vi "Auto_calibrate.vi"(3 "Mode":T4, 5 "Traverse line":T5 {"Row Duration (mins)" format="%#.1f"; "Row No" min=0; "Trace Gas Concentration (%)" min=0.0 format="%#.2f"; "Emission Rate (l/min)" format="%#.2f"; "Tunnel Speed" format="%#.2f"; "Start X" format="%#.2f"; "Start Y" format="%#.2f"; "Start Z" format="%#.2f"; "End X" format="%#.2f"; "End Y" format="%#.2f"; "End Z" format="%#.2f"; "Averaging time (min)" min=0.0 format="%#.2f"}) -> (0 "Error Messages":string, 1 "Status":T2, 2 "Traverse Out":T5 {"Row Duration (mins)" format="%#.1f"; "Row No" min=0; "Trace Gas Concentration (%)" min=0.0 format="%#.2f"; "Emission Rate (l/min)" format="%#.2f"; "Tunnel Speed" format="%#.2f"; "Start X" format="%#.2f"; "Start Y" format="%#.2f"; "Start Z" format="%#.2f"; "End X" format="%#.2f"; "End Y" format="%#.2f"; "End Z" format="%#.2f"; "Averaging time (min)" min=0.0 format="%#.2f"})   [LabVIEW 2012]
uses:
  Gen Trav/Traverse_cluster.ctl
  Gen Trav/Spacing.ctl
  Controls/Multi_run_mode.ctl
  Controls/User_Specific_mode.ctl
  Controls/Auto_Calib_Type.ctl
  Gen Trav/Multi_Run_Status.ctl
  Controls/Auto_Calib_Case.ctl
  File/Setup_Filetype.ctl
  Calibration/Calib_mode.ctl
  Controls/Setup.ctl
  Controls/Post_Process.ctl
  Controls/Save_Data.ctl
  Controls/App_Global.ctl
  Globals/Meas_global.vi
  Globals/Calib_global.vi
  Globals/Trav_pos_global.vi
  <vilib>/Analysis/baseanly.llb/Mean (DBL).vi
  Globals/Extra_Commands_Global.vi
  <vilib>/Analysis/NI_AALBase.lvlib
panel:
  out "Minimum St Dev":dbl[](array[numeric])
  out "Time FFID valve moved":dbl
  out "Wait factor":dbl
  out "Establishment time":string
  out "Orig Calib file string":string
  out "Concentrations":dbl[](array[numeric])
  out "FFID St Dev":dbl[][](array[numeric]) format="%.2f"
  in  "Clear Calib History":bool
  out "Coefficients":dbl[][](array[numeric]) format="%.2f"
  out "Currently in Case":T1
  out "Valve position":dbl format="%.2f"
  out "Currently On":i32
  out "Values":dbl[][](array[numeric]) format="%.2f"
  out "FF Indexes":i16[](array[numeric])
  out "Ch No's":i16[](array[numeric])
  out "No of Calib Points":i32
  out "Root Name":string[](array[string])
  out "Original Calib File":path
  out "Calibration varying":T3
  in  "stop":bool
  out "New Calib Filenames":path[](array[path])
  # "Specific Argument Options\n      Tunnel Speed;1;2;3;4\nOR  Traverse Position\nOR   Concentration"
  # "X           Y            Z"
  # "Start"
  # "End"
  # "X           Y            Z"
  # "Start"
  # "End"
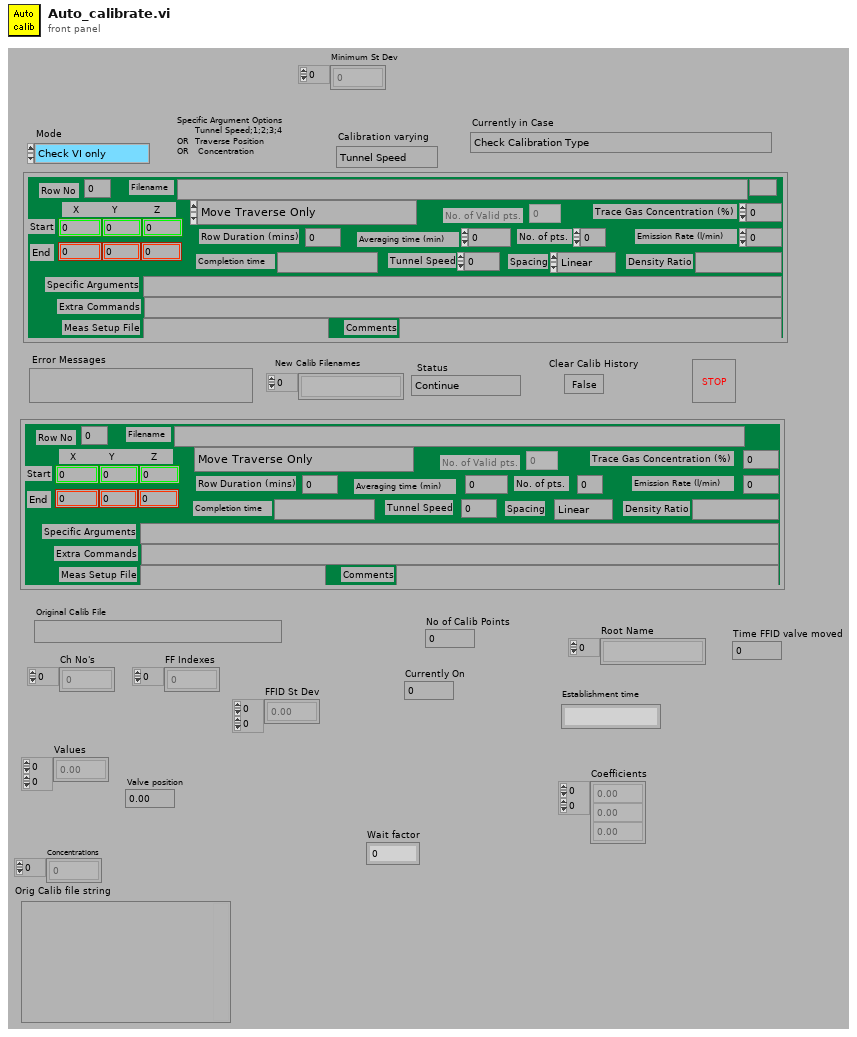
[diagram p1: front panel]
types:
  T1 = typedef "Auto_Calib_Case.ctl" = enum16{"Check Calibration Type", "Check if Original Calib file is Valid", "Get sampling rate etc. from meas setup file", "Setup Calibration Program", "Get Channel Numbers", "Check use latest selected on Mesurement setup files", "Create New Calib Filenames", "Setup Calibration Values in 2D array", "Create Measurement Setup File (Concentration Only)", "Are There Enough Calibration Points", "Set Measurement Conditions", "Measure Calibration Point", "Do Another Calibration Point?", "Skip Next Frame?", "Insert New calibration Filenames into Measurement Setup file", "Warn if FFID calibration is very non linear", "Warn if FFID variance is high", "Insert Bkgnd Variance into calib file", "Warn if FFID voltages are too low", "Warn if Current Calibration fit is poor", "Warn if Calibration Coefficients have significantly altered", "End"}
  T2 = typedef "Multi_Run_Status.ctl" = enum16{"Continue", "Jump to Next Point", "Jump to Next Row", "Jump To Fall Back", "Terminate Run"}
  T3 = typedef "Auto_Calib_Type.ctl" = enum16{"Tunnel Speed", "Traverse Position", "Concentration"}
  T4 = typedef "User_Specific_mode.ctl" = enum16{"Check VI only", "Run VI"}
  T5 = typedef "Traverse_cluster.ctl" = cluster{"Start X":dbl, "Start Y":dbl, "Start Z":dbl, "End X":dbl, "End Y":dbl, "End Z":dbl, "No. of pts.":i32, "Spacing":T6, "Filename":path, "Tunnel Speed":dbl, "Averaging time (min)":dbl, "Extra Commands":string, "Specific Arguments":string, "Emission Rate (l/min)":dbl, "Trace Gas Concentration (%)":dbl, "Density Ratio":string, "Comments":string, "Row No":i32, "Row Type Selector":T7, "Completion time":string, "Row Duration (mins)":dbl, "No. of Valid pts.":i32, "Meas Setup File":string}
  T6 = typedef "Spacing.ctl" = enum16{"Linear", "Log", "Gauss", "Specified", "N/A"}
  T7 = typedef "Multi_run_mode.ctl" = enum16{"Move Traverse Only", "Set Tunnel Speed Only", "Set Source Only", "Set Measurement Conditions", "Single Measurement", "Vertical Profile", "Lateral Profile", "Longitudinal Profile", "Explore Volume", "Multi-Axis Profile", "Auto Calibrate", "Meas Fast FID Bkgnd", "Check Beam Power", "Scanning Valve Measurement", "Run VI Named:", "Set ADAM Ch", "Wait (minutes)", "Send Message", "Synchronize With:", "Fall Back to this Row", "Turn Off Row Repeating", "Blank Row", "Traverse 3D Volume"}
  T8 = typedef "Setup_Filetype.ctl" = enum16{"Measurement Setups", "Calibration Setups", "General", "Results File Plotter Setups", "Speed Calib Tweaks"}
  T9 = typedef "Calib_mode.ctl" = enum16{"Show Setup", "Take a New Calibration Point", "Refit Curve", "Setup Front Panel"}
  T10 = typedef "Save_Data.ctl" = enum16{"Save No Data", "Save Data"}
  T11 = typedef "Post_Process.ctl" = enum16{"Take New Data", "Post Process Raw Data File"}
  T12 = typedef "Setup.ctl" = enum16{"Run Program", "Show Setup", "Save Current Setup", "Setup Front Panel"}
  T13 = typedef "App_Global.ctl" = enum16{"Read Global", "Write to Global", "Initialise Array"}
  T14 = typedef "Cal_Inst_type.ctl" = enum16{"Propeller anemometer", "Pressure Transducer", "Hot wire", "Cross wire velocity", "Cross wire angle", "Generic Linear", "Generic Polynomial", "Generic BackPoly", "Fast FID", "Thermocouple", "Cold wire", "Pulsed Wire"}
  T15 = typedef "Ref_Inst_type.ctl" = enum16{"Propellor anemometer", "Pressure Transducer", "Raw voltage", "Pitot-static tube", "Preston tube", "Generic Linear", "Generic Polynomial", "Thermocouple", "LDA", "Enter Value", "ADAM Channel"}
  T16 = cluster{"2nd Ref type":T15, "2nd inst present":bool}
  T17 = cluster{"high limit (10V)":sgl, "low limit (-10V)":sgl, "Ch No":i16, "Var name":string}[]
  T18 = cluster{"high limit (10V)":sgl, "low limit (-10V)":sgl, "Ch No":i16, "Var name":string}
  T19 = typedef "Inst_type.ctl" = enum16{"Propeller anemometer", "Raw voltage", "Pressure Transducer", "Pitot-static tube", "Preston tube", "Hot wire", "Cross wire 1", "Cross wire 2", "Generic Linear", "Generic Polynomial", "Generic BackPoly", "Fast FID", "Thermocouple", "Cold wire", "Pulsed Wire", "LDA Vel", "LDA Tran time", "LDA Arr time"}
  T20 = cluster{"high limit (10V)":sgl, "low limit (-10V)":sgl, "Ch No":i16, "Calib filename":path, "Inst type":T19, "Symbol":string, "Move channel":bool, "Use Latest":bool, "D":dbl, "Ch Name":string}[]
  T21 = typedef "Status_Cluster.ctl" = cluster{"Status":T2, "Error Type":string, "Error Description":string}
  T22 = typedef "Valco_valve_ph.ctl" = u16
  T23 = typedef "Time_Trace_Cluster.ctl" = cluster{"Weighting":dbl[], "Time (s)":dbl[], "Voltage":dbl[], "Eng Values":dbl[]}
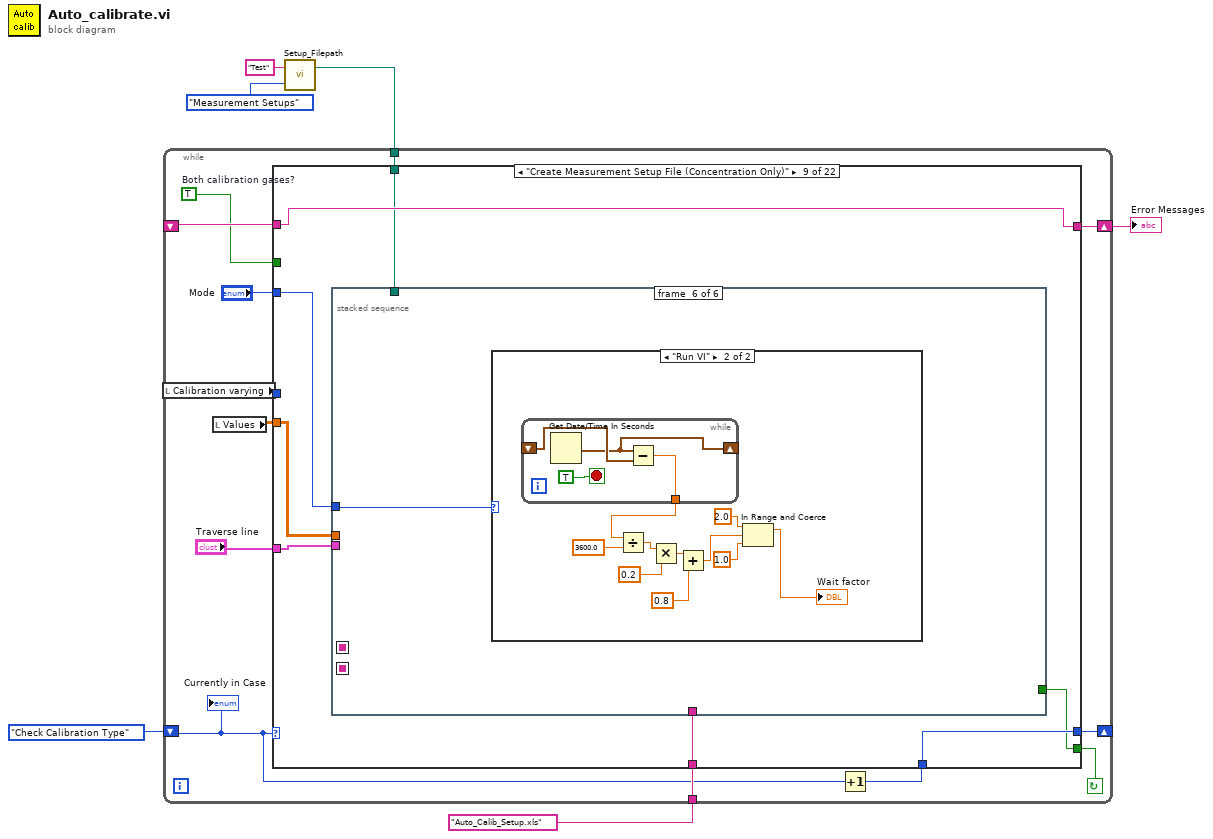
[diagram p0: block diagram]
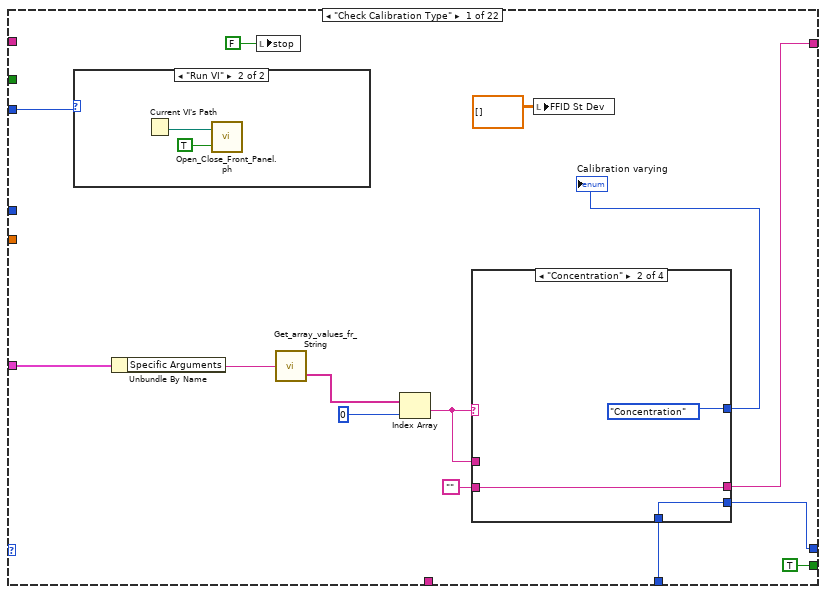
[diagram p2: hidden frame]
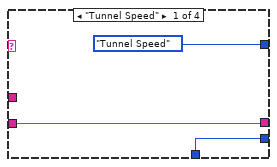
[diagram p4: hidden frame]
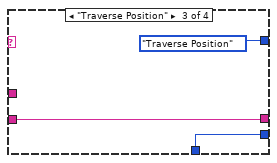
[diagram p5: hidden frame]
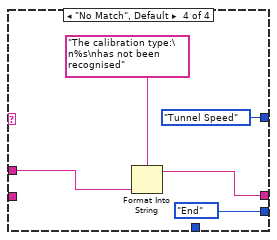
[diagram p6: hidden frame]
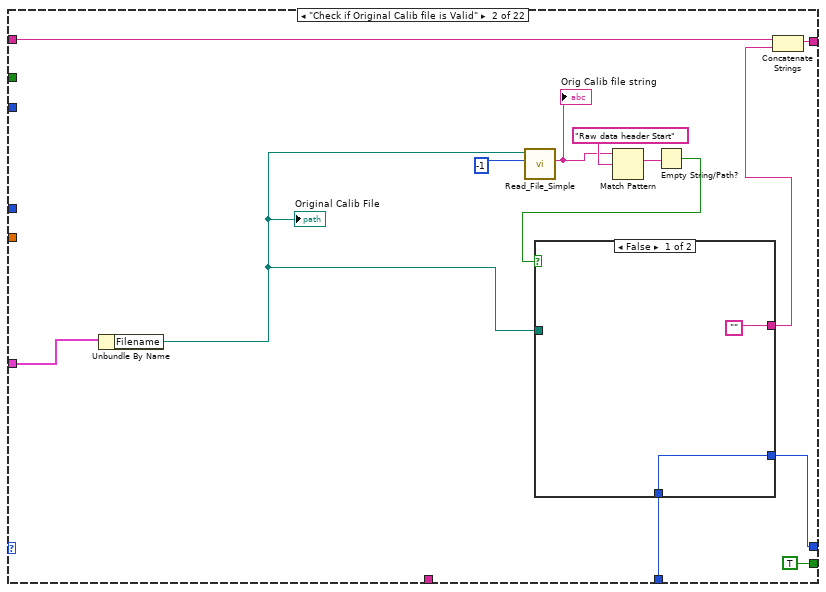
[diagram p7: hidden frame]
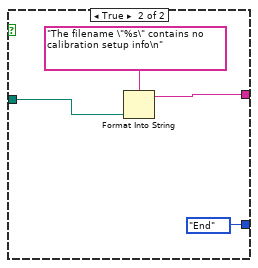
[diagram p8: hidden frame]
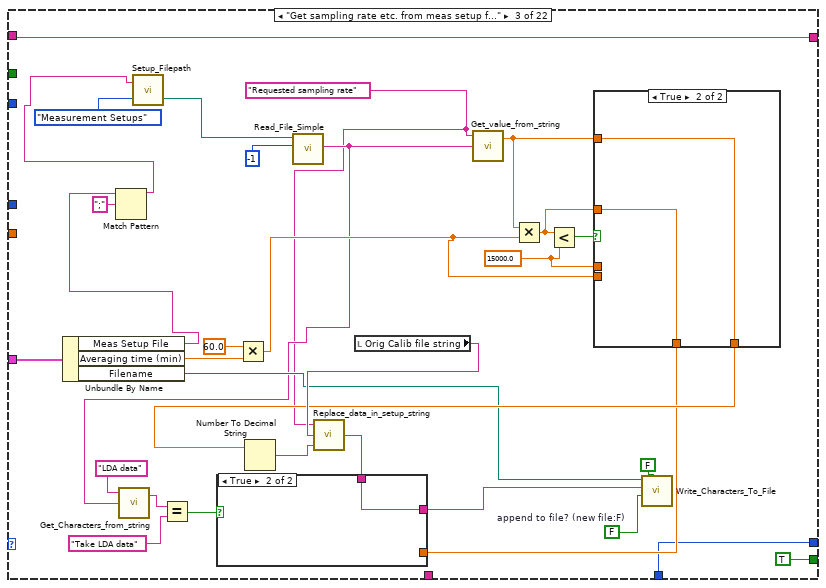
[diagram p9: hidden frame]
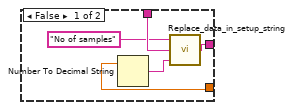
[diagram p10: hidden frame]
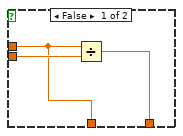
[diagram p11: hidden frame]
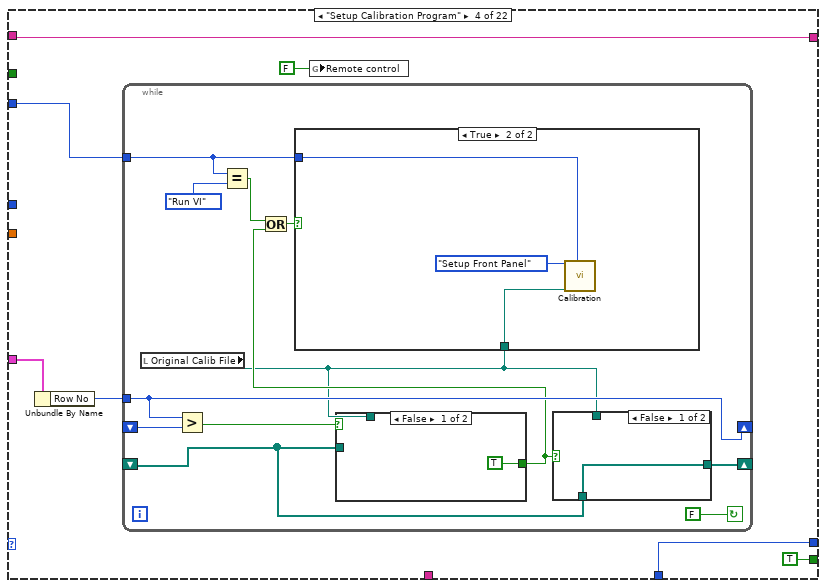
[diagram p12: hidden frame]
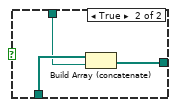
[diagram p13: hidden frame]
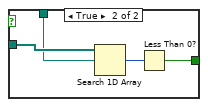
[diagram p15: hidden frame]
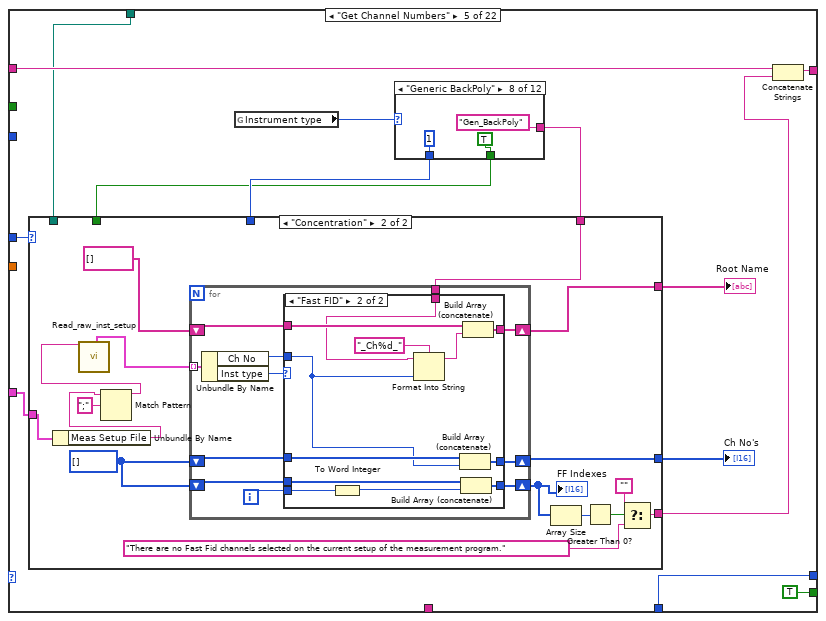
[diagram p16: hidden frame]
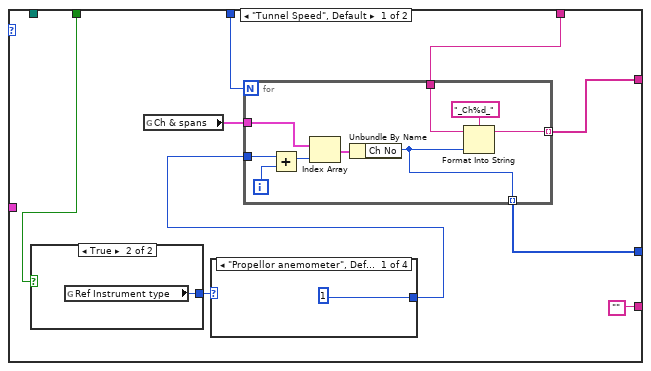
[diagram p17: hidden frame]
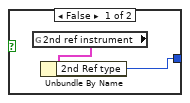
[diagram p18: hidden frame]
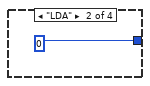
[diagram p19: hidden frame]
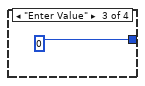
[diagram p20: hidden frame]
diagram:
  n1 = call "Setup_Filepath.vi"("Setup File Type"=Setup_Filetype."Measurement Setups", "Filename in"="Test") -> ("Directory"=w1:path)  [unwired: 1 out]
  n2 = while {
    shift-left: _ -> [w11]
    shift-right: [w12] -> w5
    shift-left: Auto_Calib_Case."Check Calibration Type" ("Currently in Case") -> [w10]
    shift-right: [w9] -> _
    tunnel: "Auto_Calib_Setup.xls" -> [w19]
    tunnel: w1 -> [w7]
    stop <- w15 continue-if-true
    w8 = TRUE  # Both calibration gases?
    n3 = local read "Calibration varying"() -> (w14:T3)
    n4 = local read "Values"() -> (w13:dbl[][])
    n5 = Increment(x=w10) -> (x+1=w16:T1)
    n6 = case shown="\"Create Measurement Setup File (Concentration Only)\"" w10 {
      tunnel: "Traverse line" -> [w33 w62 w100 w114 w145 _ _ w367 w400 _ w553 _ _ _ _ _ _ _ _ _ w970 w1001]
      tunnel: "Mode" -> [w24 _ _ w115 _ _ w318 _ w401 _ w548 _ w714 _ _ _ _ _ _ _ _ w1002]
      tunnel: w19 -> [_ _ _ _ _ _ _ _ w405 _ _ w625 _ _ _ _ _ _ _ _ _ _]
      tunnel: [w22 w52 w82 w117 w148 w264 w315 w358 w403 w516 w541 w624 w715 w741 w753 w772 w810 w875 w893 w949 w993 w1007] -> w9
      tunnel: w16 -> [w23 w51 w82 w117 w148 w264 w315 w359 w403 w515 w535 w624 _ w740 w752 w772 w810 w875 w893 w949 w993 w1007]
      tunnel: [TRUE TRUE TRUE TRUE TRUE TRUE TRUE TRUE w399 TRUE TRUE TRUE TRUE TRUE TRUE TRUE TRUE TRUE TRUE TRUE TRUE FALSE] -> w15
      tunnel: w14 -> [_ _ _ _ w152 _ w314 w365 _ _ w539 w626 w713 w739 w755 _ _ _ _ _ _ w1003]
      tunnel: w13 -> [_ _ _ _ _ _ _ _ w398 w525 w552 _ _ _ _ _ w817 _ w899 _ _ _]
      tunnel: [w26 w54 w80 w118 w149 w265 w329 w362 w404 w519 w536 w622 w712 w744 w759 w781 w824 w871 w900 w938 w986 w1006] -> w12
      tunnel: w11 -> [_ w56 w80 w118 w151 w265 w329 w361 w404 w520 w536 w622 w712 w744 w759 w781 w824 w871 w900 w938 w986 w1006]
      tunnel: w8 -> [_ _ _ _ _ _ _ w360 _ _ _ _ _ _ _ _ _ _ _ _ _ w1000]
      tunnel: w7 -> [_ _ _ _ w144 w267 _ _ w402 _ _ _ _ _ _ _ _ _ _ _ _ _]
      frame "Check Calibration Type" {
        n7 = case shown="\"Run VI\"" w24 {
          frame "Check VI only" {
          }
          frame "Run VI" {
            n8 = Current VI's Path() -> (path=w34:path)
            n9 = call "Open_Close_Front_Panel.ph.vi"("Front Panel Window:Open"=TRUE, "VI path"=w34) -> ()  [unwired: 2 out]
          }
        }
        n10 = Unbundle By Name(w33) -> ("Specific Arguments"=w32:string)
        n11 = local write "stop"(FALSE) -> ()
        n12 = call "Get_array_values_fr_String.vi"("String Value"=w32) -> ("String array"=w31:string[])  [unwired: 1 out]
        n13 = Index Array(array=w31, index=0 ("Index")) -> (element=w29:string)
        n14 = case shown="\"Concentration\"" w29 {
          tunnel: [Auto_Calib_Type."Tunnel Speed" ("Calibration varying") Auto_Calib_Type."Concentration" ("Calibration varying") Auto_Calib_Type."Traverse Position" ("Calibration varying") Auto_Calib_Type."Tunnel Speed" ("Calibration varying")] -> w27
          tunnel: w29 -> [_ _ _ w48]
          tunnel: [w37 w40 w43 w46] -> w26
          tunnel: "" -> [w37 w40 w43 _]
          tunnel: w23 -> [w36 w39 w42 _]
          tunnel: [w36 w39 w42 Auto_Calib_Case."End" ("Currently in Case")] -> w22
          frame "Tunnel Speed" {
          }
          frame "Concentration" {
            (unwired) ""
          }
          frame "Traverse Position" {
          }
          frame "No Match", Default {
            n15 = Format Into String(format string="The calibration type:\n%s\nhas not been recognised" ("Format String"), w48) -> (resulting string=w46:string)  [unwired: 2 in, 1 out]
          }
        }
        "Calibration varying" <- w27
        n16 = local write "FFID St Dev"(dbl[][] [] ("FFID Variance")) -> ()
      }
      frame "Check if Original Calib file is Valid" {
        n17 = Unbundle By Name(w62) -> ("Filename"=w50:path)
        "Original Calib File" <- w50
        n18 = call "Read_File_Simple.vi"("Filename"=w50, "number of characters (all:-1)"=-1) -> ("string"=w59:string)  [unwired: 1 in, 7 out]
        "Orig Calib file string" <- w59
        n19 = Match Pattern(string=w59, regular expression="Raw data header Start") -> (match substring=w58:string)  [unwired: 4 out]
        n20 = Empty String/Path?(string/path=w58) -> (empty?=w57:bool)
        n21 = case shown="False" w57 {
          tunnel: w50 -> [_ w68]
          tunnel: ["" w66] -> w55
          tunnel: [w63 Auto_Calib_Case."End" ("Currently in Case")] -> w52
          tunnel: w51 -> [w63 _]
          frame False {
          }
          frame True {
            n22 = Format Into String(format string="The filename \"%s\" contains no calibration setup info\n" ("Format String"), w68) -> (resulting string=w66:string)  [unwired: 2 in, 1 out]
          }
        }
        n23 = Concatenate Strings(w56, w55) -> (w54:string)
      }
      frame "Get sampling rate etc. from meas setup file" {
        w83 = FALSE  # append to file? (new file:F)
        w72 = "Requested sampling rate"
        w90 = 15000.0 ("y")
        n24 = Unbundle By Name(w100) -> ("Meas Setup File"=w78:string, "Averaging time (min)"=w98:dbl, "Filename"=w85:path)
        n25 = Match Pattern(string=w78, regular expression=";") -> (before substring=w70:string)  [unwired: 4 out]
        n26 = call "Setup_Filepath.vi"("Setup File Type"=Setup_Filetype."Measurement Setups", "Filename in"=w70) -> ("Filename Out"=w69:path)  [unwired: 1 out]
        n27 = Multiply(x=60.0, y=w98) -> (x*y=w89:dbl)
        n28 = call "Read_File_Simple.vi"("Filename"=w69, "number of characters (all:-1)"=-1) -> ("string"=w77:string)  [unwired: 1 in, 7 out]
        n29 = call "Get_Characters_from_string.vi"("Input string"=w77, "Variable name"="LDA data") -> ("Value"=w75:string)  [unwired: 1 in, 1 out]
        n30 = Equal?(x=w75, y="Take LDA data") -> (x = y?=w73:bool)
        n31 = local read "Orig Calib file string"() -> (w94:string)
        n32 = call "Get_value_from_string.vi"("Input string"=w77, "Variable name"=w72) -> ("Value"=w93:dbl)  [unwired: 1 in, 1 out]
        n33 = Multiply(x=w93, y=w89) -> (x*y=w88:dbl)
        n34 = Less?(x=w88, y=w90) -> (x < y?=w96:bool)
        n35 = case shown="True" w96 {
          tunnel: w93 -> [_ w111]
          tunnel: [w108 w111] -> w92
          tunnel: w90 -> [w107 _]
          tunnel: w89 -> [w109 _]
          tunnel: [w107 w110] -> w86
          tunnel: w88 -> [_ w110]
          frame False {
            n36 = Divide(x=w107, y=w109) -> (x/y=w108:dbl)
          }
          frame True {
          }
        }
        n37 = Number To Decimal String(number=w92) -> (decimal integer string=w91:string)  [unwired: 1 out]
        n38 = call "Replace_data_in_setup_string.vi"("New data string"=w91, "Input string"=w94, "Variable name"=w72) -> ("Appended string"=w87:string)
        n39 = case shown="True" w73 {
          tunnel: w87 -> [w105 w106]
          tunnel: w86 -> [w102 _]
          tunnel: [w101 w106] -> w84
          frame False {
            n40 = Number To Decimal String(number=w102) -> (decimal integer string=w103:string)  [unwired: 1 out]
            n41 = call "Replace_data_in_setup_string.vi"("New data string"=w103, "Input string"=w105, "Variable name"="No of samples") -> ("Appended string"=w101:string)
          }
          frame True {
          }
        }
        n42 = call "Write_Characters_To_File.vi"("file path (dialog if empty)"=w85, "advisory dialog? (display:T)"=FALSE, "character string"=w84, "append to file? (new file:F)"=w83) -> ()  [unwired: 1 in, 4 out]
      }
      frame "Setup Calibration Program" {
        n43 = Unbundle By Name(w114) -> ("Row No"=w113:i32)
        n44 = while {
          shift-left: _ -> [w122]
          shift-right: [w120] -> _
          tunnel: w113 -> [w129]
          shift-left: _ -> [w130]
          shift-right: [w129] -> _
          tunnel: w115 -> [w127]
          stop <- FALSE continue-if-true
          n45 = local read "Original Calib File"() -> (w121:path)
          n46 = Greater?(x=w129, y=w130) -> (0:w128:bool)
          n47 = Equal?(x=w127, y=User_Specific_mode."Run VI" ("Mode")) -> (x = y?=w125:bool)
          n48 = case shown="False" w128 {
            tunnel: w122 -> [_ w142]
            tunnel: w121 -> [_ w141]
            tunnel: [TRUE w139] -> w123
            frame False {
            }
            frame True {
              n49 = Search 1D Array(1D array=w142, element=w141) -> (index of element=w140:i32)  [unwired: 1 out]
              n50 = Less Than 0?(x=w140) -> (x < 0?=w139:bool)
            }
          }
          n51 = Or(x=w125, y=w123) -> (x .or. y?=w124:bool)
          n52 = case shown="True" w124 {
            tunnel: w127 -> [_ w137]
            tunnel: w121 -> [_ w136]
            frame False {
            }
            frame True {
              n53 = call "Calibration.vi"("Mode"=Calib_mode."Setup Front Panel", "Calib file"=w136, "Simulate/Run"=w137) -> ()  [unwired: 17 out]
            }
          }
          n54 = case shown="False" w123 {
            tunnel: w122 -> [w131 w134]
            tunnel: w121 -> [_ w133]
            tunnel: [w131 w132] -> w120
            frame False {
            }
            frame True {
              n55 = Build Array (concatenate)(w134, w133) -> (w132:path[])
            }
          }
        }
        n56 = global write "Meas_global.vi" "Remote control"(FALSE ("Remote control")) -> ()
      }
      frame "Get Channel Numbers" {
        n57 = global read "Calib_global.vi" "Instrument type"() -> (w156:T14)
        n58 = case shown="\"Generic BackPoly\"" w156 {
          tunnel: ["Prop" "Mano" "HW" "XW" "XW" "Gen_Lin" "Gen_Poly" "Gen_BackPoly" "FF" "Therm" "CW" "PWA"] -> w155
          tunnel: [1 1 1 2 2 1 1 1 1 1 1 1] -> w146
          tunnel: [TRUE TRUE TRUE TRUE FALSE TRUE TRUE TRUE TRUE TRUE TRUE TRUE] -> w143
          frame "Propeller anemometer" {
          }
          frame "Pressure Transducer" {
          }
          frame "Hot wire" {
          }
          frame "Cross wire velocity" {
          }
          frame "Cross wire angle" {
          }
          frame "Generic Linear" {
          }
          frame "Generic Polynomial" {
          }
          frame "Generic BackPoly" {
          }
          frame "Fast FID" {
          }
          frame "Thermocouple" {
          }
          frame "Cold wire" {
          }
          frame "Pulsed Wire" {
          }
        }
        n59 = case shown="\"Concentration\"" w152 {
          tunnel: w155 -> [w163 w197]
          tunnel: [w159 w196] -> w154
          tunnel: [w160 w194] -> w153
          tunnel: ["" w187] -> w150
          tunnel: w146 -> [w161 _]
          tunnel: w145 -> [_ w186]
          tunnel: w144 -> [_ _]
          tunnel: w143 -> [w157 _]
          frame "Tunnel Speed", Default {
            n60 = case shown="True" w157 {
              tunnel: [w166 w168] -> w165
              frame False {
                n61 = global read "Calib_global.vi" "2nd ref instrument"() -> (w167:T16)
                n62 = Unbundle By Name(w167) -> ("2nd Ref type"=w166:T15)
              }
              frame True {
                n63 = global read "Calib_global.vi" "Ref Instrument type"() -> (w168:T15)
              }
            }
            n64 = global read "Calib_global.vi" "Ch & spans"() -> (w162:T17)
            n65 = case shown="\"Propellor anemometer\", Default" w165 {
              tunnel: [1 i16 0 0 0] -> w158
              frame "Propellor anemometer", Default {
              }
              frame "LDA" {
              }
              frame "Enter Value" {
              }
              frame "ADAM Channel" {
              }
            }
            n66 = for {
              N: w161 -> [_]
              tunnel: [w175] -> w160 mode=indexing
              tunnel: w163 -> [w174]
              tunnel: w162 -> [w173]
              tunnel: [w172] -> w159 mode=indexing
              tunnel: w158 -> [w170]
              i -> [w171]
              n67 = Add(x=w170, y=w171) -> (x+y=w169:i32)
              n68 = Index Array(array=w173, index=w169) -> (element=w177:T18)
              n69 = Unbundle By Name(w177) -> ("Ch No"=w175:i16)
              n70 = Format Into String(format string="_Ch%d_" ("Format String"), initial string=w174, w175) -> (resulting string=w172:string)  [unwired: 1 in, 1 out]
            }
          }
          frame "Concentration" {
            w193 = i16[] []
            n71 = Unbundle By Name(w186) -> ("Meas Setup File"=w183:string)
            n72 = Match Pattern(string=w183, regular expression=";") -> (before substring=w182:string)  [unwired: 4 out]
            n73 = call "Read_raw_inst_setup.vi"("Setup file"=w182) -> ("Ch & spans choices"=w185:T20)  [unwired: 18 out]
            n74 = for {
              tunnel: w185 -> [w208] mode=indexing
              tunnel: w197 -> [w207]
              shift-right: [w203] -> w196
              shift-left: string[] [] -> [w204]
              shift-right: [w201] -> w194
              shift-left: w193 -> [w202]
              shift-right: [w200] -> w192
              shift-left: w193 -> [w199]
              i -> [w198]
              n75 = Unbundle By Name(w208) -> ("Ch No"=w206:i16, "Inst type"=w205:T19)
              n76 = case shown="\"Fast FID\"" w205 {
                tunnel: w207 -> [_ w213]
                tunnel: w206 -> [_ w215]
                tunnel: w204 -> [w211 w223]
                tunnel: [w211 w222] -> w203
                tunnel: w202 -> [w210 w221]
                tunnel: [w210 w220] -> w201
                tunnel: w199 -> [w209 w218]
                tunnel: [w209 w219] -> w200
                tunnel: w198 -> [_ w217]
                frame "Generic Linear", Default {
                }
                frame "Fast FID" {
                  n77 = To Word Integer(number=w217) -> (16bit integer=w216:i16)
                  n78 = Format Into String(format string="_Ch%d_", initial string=w213, w215) -> (resulting string=w212:string)  [unwired: 1 in, 1 out]
                  n79 = Build Array (concatenate)(w221, w215) -> (w220:i16[])
                  n80 = Build Array (concatenate)(w218, w216) -> (w219:i16[])
                  n81 = Build Array (concatenate)(w223, w212) -> (w222:string[])
                }
              }
            }
            "FF Indexes" <- w192
            n82 = Array Size(array=w192) -> (size(s)=w191:i32)
            n83 = Greater Than 0?(x=w191) -> (x > 0?=w190:bool)
            n84 = Select(t="", s=w190, f="There are no Fast Fid channels selected on the current setup of the measurement program.") -> (s? t:f=w187:string)
          }
        }
        "Root Name" <- w154
        "Ch No's" <- w153
        n85 = Concatenate Strings(w151, w150) -> (w149:string)
      }
      frame "Check use latest selected on Mesurement setup files" {
        n86 = global read "Trav_pos_global.vi" "Measurement setup files"() -> (w260:string[])
        n87 = local read "Ch No's"() -> (w266:i16[])
        n88 = Build Array (concatenate)(w260, "Current_Setup.xls") -> (w261:string[])
        n89 = for {
          tunnel: w267 -> [w270]
          tunnel: w261 -> [w269] mode=indexing
          tunnel: w266 -> [w268]
          n90 = stacked-sequence {
            seq-local: [w271 _ _] -> [_ w277 w305]
            seq-local: [_ w275 _] -> [_ _ w303]
            tunnel: w270 -> [w274 _ w302]
            tunnel: w269 -> [w273 _ w301]
            tunnel: w268 -> [_ w276 _]
            frame #0 {
              n91 = Build Path(base path=w274, name or relative path=w273) -> (appended path=w272:path)
              n92 = call "Read_File_Simple.vi"("Filename"=w272) -> ("string"=w271:string)  [unwired: 2 in, 7 out]
            }
            frame #1 {
              n93 = while {
                shift-right: [w282] -> w275
                shift-left: w277 -> [w283]
                tunnel: w276 -> [w286]
                i -> [w290]
                stop <- w279 continue-if-true
                n94 = Increment(x=w290) -> (x+1=w284:i32)
                n95 = Format Into String(format string="An ch %d Ch No", w284) -> (resulting string=w289:string)  [unwired: 2 in, 1 out]
                n96 = call "Get_value_from_string.vi"("Input string"=w283, "Variable name"=w289) -> ("Status"=w288:enum16{"Char in string", "Char not in string"}, "Value"=w287:dbl)  [unwired: 1 in]
                n97 = To Long Integer(number=w287) -> (32bit integer=w285:i32)
                n98 = Search 1D Array(1D array=w286, element=w285) -> (index of element=w281:i32)  [unwired: 1 in]
                n99 = Greater Or Equal To 0?(x=w281) -> (x >= 0?=w280:bool)
                n100 = case shown="\"Char in string\"" w288 {
                  tunnel: [TRUE FALSE] -> w279
                  frame "Char in string" {
                  }
                  frame "Char not in string" {
                  }
                }
                n101 = And(x=w280, y=w279) -> (x .and. y?=w278:bool)
                n102 = case shown="True" w278 {
                  tunnel: w284 -> [w294 _]
                  tunnel: w283 -> [w293 w298]
                  tunnel: [w292 w298] -> w282
                  frame True {
                    n103 = Format Into String(format string="An ch %d Use latest Calib", w294) -> (resulting string=w296:string)  [unwired: 2 in, 1 out]
                    n104 = call "Replace_data_in_setup_string.vi"("New data string"="TRUE" ("Replace with"), "Input string"=w293, "Variable name"=w296) -> ("Appended string"=w292:string)
                  }
                  frame False {
                  }
                }
              }
            }
            frame #2 {
              n105 = Equal?(x=w305, y=w303) -> (x = y?=w304:bool)
              n106 = case shown="True" w304 {
                tunnel: w302 -> [w308 _]
                tunnel: w303 -> [w311 _]
                tunnel: w301 -> [w307 _]
                frame False {
                  w310 = FALSE  # append to file? (new file:F)
                  n107 = Build Path(base path=w308, name or relative path=w307) -> (appended path=w306:path)
                  n108 = call "Write_Characters_To_File.vi"("file path (dialog if empty)"=w306, "advisory dialog? (display:T)"=FALSE, "character string"=w311, "append to file? (new file:F)"=w310) -> ()  [unwired: 1 in, 4 out]
                }
                frame True {
                }
              }
            }
          }
        }
      }
      frame "Create New Calib Filenames" {
        n109 = local read "Original Calib File"() -> (w327:path)
        n110 = Get Date/Time String(date format (0)=enum16{"short", "long", "abbreviated"}."short") -> (date string=w322:string)  [unwired: 3 out]
        n111 = Strip Path(path=w327) -> (stripped path=w317:path)  [unwired: 1 out]
        n112 = local read "Root Name"() -> (w313:string[])
        n113 = case shown="\"Tunnel Speed\", Default" w314 {
          tunnel: w313 -> [_ w334]
          tunnel: [1 w333] -> w312
          frame "Tunnel Speed", Default {
          }
          frame "Concentration" {
            n114 = Array Size(array=w334) -> (size(s)=w333:i32)
          }
        }
        n115 = call "Replace_Character.vi"("Replace with"="-", "Input String"=w322, "Search For"="/") -> ("Output string"=w319:string)  [unwired: 1 out]
        n116 = List Folder(path=w317) -> (filenames=w331:string[])  [unwired: 1 in, 5 out]
        n117 = To Upper Case(1:w331) -> (0:w330:string[])
        n118 = for {
          N: w312 -> [_]
          tunnel: w313 -> [w337] mode=indexing
          tunnel: w330 -> [w341]
          tunnel: w317 -> [w340]
          tunnel: [w336] -> w326 mode=indexing
          tunnel: w319 -> [w338]
          tunnel: w318 -> [w335]
          n119 = while {
            tunnel: w337 -> [w348]
            tunnel: w338 -> [w349]
            tunnel: [w344] -> w339
            tunnel: w341 -> [w351]
            i -> [w353]
            stop <- w355 continue-if-true
            n120 = Increment(x=w353) -> (x+1=w350:i32)
            n121 = Format Into String(format string="%s_%d.xls" ("Format String"), initial string=w348, w349, w350) -> (resulting string=w345:string)  [unwired: 1 in, 1 out]
            n122 = call "Replace_Character.vi"("Replace with"="_", "Input String"=w345, "Search For"=" ") -> ("Output string"=w344:string)  [unwired: 1 out]
            n123 = To Upper Case(1:w344) -> (0:w354:string)
            n124 = Search 1D Array(1D array=w351, element=w354) -> (index of element=w356:i32)  [unwired: 1 out]
            n125 = Not Equal?(x=w356, y=-1) -> (x != y?=w355:bool)
          }
          n126 = Build Path(base path=w340, name or relative path=w339) -> (appended path=w336:path)
          n127 = case shown="\"Run VI\"" w335 {
            tunnel: w336 -> [_ w342]
            frame "Check VI only" {
            }
            frame "Run VI" {
              n128 = call "Calibration.vi"("Mode"=Calib_mode."Setup Front Panel", "Calib file"=w342) -> ()  [unwired: 1 in, 17 out]
            }
          }
        }
        "New Calib Filenames" <- w326
        n129 = Index Array(array=w326, index=0 ("Index")) -> (element=w324:path)
        n130 = global write "Meas_global.vi" "Results file"(w324) -> ()
        "Establishment time" <- "!Establish Exp Conditions (s) = 15" ("Message")
      }
      frame "Setup Calibration Values in 2D array" {
        n131 = case shown="\"Concentration\"" w365 {
          tunnel: [w376 w382 w397] -> w364
          tunnel: w367 -> [w371 _ w396]
          tunnel: ["" "" w395] -> w363
          tunnel: w360 -> [_ w380 _]
          tunnel: w359 -> [w370 w379 w394]
          tunnel: [w369 w379 w393] -> w358
          frame "Tunnel Speed" {
            n132 = Unbundle By Name(w371) -> ("Specific Arguments"=w374:string)
            n133 = call "Get_array_values_fr_String.vi"("String Value"=w374) -> ("Numeric Array"=w372:dbl[])  [unwired: 1 out]
            n134 = Array Subset(array=w372, index=1 ("Array Index")) -> (w368:dbl[])  [unwired: 1 in]
            n135 = for {
              tunnel: w368 -> [w378] mode=indexing
              tunnel: [w377] -> w376 mode=indexing
              n136 = Build Array(w378) -> (w377:dbl[])
            }
            n137 = Increment(x=w370) -> (x+1=w369:T1)
          }
          frame "Concentration" {
            n138 = case shown="True" w380 {
              tunnel: [w384 w388] -> w383
              frame True {
                n139 = Build Array(3.0, 2.0, 1.0) -> (w384:dbl[])
              }
              frame False {
                n140 = Build Array(1.0, 3.0) -> (w388:dbl[])
              }
            }
            n141 = for {
              tunnel: w383 -> [w392] mode=indexing
              tunnel: [w391] -> w382 mode=indexing
              n142 = Build Array(w392) -> (w391:dbl[])
            }
          }
          frame "Traverse Position" {
            n143 = call "Create_Pos_array.vi"("Traverse line"=w396) -> ("Error Messages"=w395:string, "Array of Positions"=w397:dbl[][])  [unwired: 5 in, 2 out]
            n144 = Increment(x=w394) -> (x+1=w393:T1)
          }
        }
        "Values" <- w364
        n145 = Concatenate Strings(w361, w363) -> (w362:string)
      }
      frame "Create Measurement Setup File (Concentration Only)" {
        n146 = stacked-sequence {
          seq-local: [w416 _ _ _ _ _] -> [_ w435 _ _ _ _]
          seq-local: [_ w433 _ _ _ _] -> [_ _ w456 _ _ _]
          tunnel: w402 -> [w407 _ w457 _ _ _]
          tunnel: w405 -> [_ _ w458 _ _ _]
          tunnel: w401 -> [_ _ _ w464 w483 w500]
          tunnel: w400 -> [w413 _ _ _ w484 _]
          tunnel: [_ _ _ _ w482 _] -> w399
          tunnel: w398 -> [_ _ _ w467 _ _]
          frame #0 {
            w420 = TRUE  # Show Dialog?
            n147 = Unbundle By Name(w413) -> ("Meas Setup File"=w414:string)
            n148 = Match Pattern(string=w414, regular expression=";") -> (before substring=w412:string)  [unwired: 4 out]
            n149 = Build Path(base path=w407, name or relative path=w412) -> (appended path=w421:path)
            n150 = Format Into String(format string="Meas Setup File   %s", w407) -> (resulting string=w406:string)  [unwired: 2 in, 1 out]
            n151 = call "Read_spec_No_of_Characters.vi"("Filename"=w421) -> ("character string"=w422:string)  [unwired: 1 out]
            n152 = call "Get_string_subset.vi"("String Name"=w406, "Show Dialog?"=w420, "String to split"=w422, "File Label"="Raw data header") -> ("Output string"=w409:string)  [unwired: 1 out]
            n153 = call "Get_value_from_string.vi"("Input string"=w409, "Variable name"="No of analogue inst") -> ("Value"=w410:dbl)  [unwired: 1 in, 1 out]
            n154 = for {
              N: w410 -> [_]
              shift-right: [w424] -> w419
              shift-left: w409 -> [w426]
              i -> [w430]
              n155 = Increment(x=w430) -> (x+1=w429:i32)
              n156 = Number To Decimal String(number=w429) -> (decimal integer string=w432:string)  [unwired: 1 out]
              n157 = Concatenate Strings("An ch ", w432, " Inst type") -> (w427:string)
              n158 = call "Replace_data_in_setup_string.vi"("New data string"="Raw voltage", "Input string"=w426, "Variable name"=w427) -> ("Appended string"=w424:string)
            }
            n159 = call "Replace_data_in_setup_string.vi"("New data string"="No LDA data", "Input string"=w419, "Variable name"="LDA data" ("Label for characters")) -> ("Appended string"=w416:string)
          }
          frame #1 {
            n160 = global read "Calib_global.vi" "New Setup String"() -> (w436:string)
            n161 = for {
              N: 4 -> [_]
              shift-right: [w441] -> w433
              shift-left: w435 -> [w442]
              tunnel: w436 -> [w438]
              i -> [w440]
              n162 = case shown="3" w440 {
                tunnel: [w445 w448 w451 "No of blocks"] -> w439
                tunnel: w438 -> [w444 w447 w450 _]
                tunnel: [w443 w446 w449 "1" ("Value")] -> w437
                frame 0, Default {
                  w445 = "No of samples"
                  n163 = call "Get_Characters_from_string.vi"("Input string"=w444, "Variable name"=w445) -> ("Value"=w443:string)  [unwired: 1 in, 1 out]
                }
                frame 2 {
                  w448 = "Actual sampling rate"
                  n164 = call "Get_Characters_from_string.vi"("Input string"=w447, "Variable name"=w448) -> ("Value"=w446:string)  [unwired: 1 in, 1 out]
                }
                frame 3 {
                  w451 = "Board type"
                  n165 = call "Get_Characters_from_string.vi"("Input string"=w450, "Variable name"=w451) -> ("Value"=w449:string)  [unwired: 1 in, 1 out]
                }
                frame 1 {
                }
              }
              n166 = call "Replace_data_in_setup_string.vi"("New data string"=w437, "Input string"=w442, "Variable name"=w439) -> ("Appended string"=w441:string)
            }
          }
          frame #2 {
            w462 = FALSE  # advisory dialog? (display:T)
            w463 = FALSE  # append to file? (new file:F)
            n167 = call "Remove_Plug_Ins_etc.vi"("Input String"=w456) -> ("Output string"=w455:string)
            n168 = call "Add_label_to_string.vi"("String to write"=w455, "File Label"="Raw data header") -> ("Output string"=w459:string)
            n169 = Build Path(base path=w457, name or relative path=w458) -> (appended path=w454:path)
            n170 = call "Add_length_to_string.vi"("String in"=w459) -> ("String out"=w461:string)
            n171 = call "Write_Characters_To_File.vi"("file path (dialog if empty)"=w454, "advisory dialog? (display:T)"=w462, "character string"=w461, "append to file? (new file:F)"=w463) -> ()  [unwired: 1 in, 4 out]
          }
          frame #3 {
            w466 = 0 ("Index")
            w471 = 0.0 ("Input Element")
            n172 = Index Array(array=w467, index (row)=w466, index (col)=w466) -> (element=w465:dbl)
            n173 = case shown="\"Run VI\"" w464 {
              tunnel: w465 -> [_ w474]
              frame "Check VI only" {
              }
              frame "Run VI" {
                n174 = flat-sequence {
                  tunnel: w474 -> [w475]
                  frame #0 {
                    n175 = call "Fast_FID_Valve_Control.vi"("Requested Position"=w475) -> ()  [unwired: 7 out]
                  }
                  frame #1 {
                    n176 = Get Date/Time In Seconds() -> (seconds since 1Jan1904=w477:timestamp)
                    n177 = To Double Precision Float(number=w477) -> (double precision float=→"Time FFID valve moved":dbl)
                  }
                }
              }
            }
            n178 = Build Array("GMU:Calibration:Gas 1", "GMU:Calibration:Gas 2") -> (w473:string[])
            n179 = call "Get_Current_Scan_client.vi"("ADAM Ch Names"=w473) -> ("Numerical Values"=w472:dbl[])  [unwired: 3 out]
            n180 = Build Array (concatenate)(w471, w471, w472, w471) -> (→"Concentrations":dbl[])
          }
          frame #4 {
            w481 = dbl[] [30.0, 15.0, 0.0] ("appended array")
            n181 = Unbundle By Name(w484) -> ("Start Z"=w478:dbl)
            n182 = Array Size(array=w481) -> (size(s)=w480:i32)
            n183 = Decrement(x=w480) -> (x-1=w479:i32)
            n184 = while {
              tunnel: w483 -> [w493]
              tunnel: w484 -> [w497]
              tunnel: w481 -> [w496] mode=indexing
              tunnel: w478 -> [w494]
              tunnel: w479 -> [w489]
              tunnel: [w485] -> w482
              i -> [w490]
              stop <- w486 continue-if-true
              n185 = Add(x=w494, y=w496) -> (x+y=w495:dbl)
              n186 = Less?(x=w490, y=w489) -> (x < y?=w487:bool)
              n187 = Bundle By Name(cluster=w497, "Start Z"=w495) -> (w498:T5)
              n188 = call "Set_Traverse_Position.vi"("Simulate/Run"=w493, "Currently on Point"=1, "Traverse line"=w498) -> ("Status Cluster"=w488:T21)  [unwired: 2 out]
              n189 = Unbundle By Name(w488) -> ("Status"=w491:T2)
              n190 = call "Prog_Status_Handler.vi"("Status Cluster"=w488, "Simulate/Run"=w493) -> ()  [unwired: 2 out]
              n191 = local write "Status"(w491) -> ()
              n192 = Equal?(x=w491, y=Multi_Run_Status."Continue" ("Status")) -> (x = y?=w485:bool)
              n193 = And(x=w485, y=w487) -> (x .and. y?=w486:bool)
            }
          }
          frame #5 {
            n194 = case shown="\"Run VI\"" w500 {
              frame "Check VI only", Default {
              }
              frame "Run VI" {
                n195 = while {
                  shift-right: [w512] -> _
                  shift-left: _ -> [w513]
                  tunnel: [w511] -> w506
                  stop <- TRUE stop-if-true
                  n196 = Get Date/Time In Seconds() -> (seconds since 1Jan1904=w512:timestamp)
                  n197 = Subtract(x=w512, y=w513) -> (x-y=w511:dbl)
                }
                n198 = Divide(x=w506, y=3600.0) -> (x/y=w505:dbl)
                n199 = Multiply(x=w505, y=0.2) -> (x*y=w503:dbl)
                n200 = Add(x=w503, y=0.8) -> (x+y=w501:dbl)
                n201 = In Range and Coerce(upper limit=2.0, x=w501, lower limit=1.0) -> (coerced(x)=→"Wait factor":dbl)  [unwired: 1 out]
              }
            }
          }
        }
      }
      frame "Are There Enough Calibration Points" {
        n202 = Array Size(array=w525) -> (size(s)=w526:i32[])
        n203 = Index Array(array=w526, index=0 ("Index")) -> (element=w521:i32)
        "No of Calib Points" <- w521
        n204 = Greater?(x=w521, y=1) -> (0:w522:bool)
        n205 = case shown="False" w522 {
          tunnel: ["Less than two calibration points have been specified\n" ""] -> w518
          tunnel: [Auto_Calib_Case."End" ("Currently in Case") w530] -> w516
          tunnel: w515 -> [_ w530]
          frame False {
          }
          frame True {
          }
        }
        n206 = Concatenate Strings(w520, w518) -> (w519:string)
        "Currently On" <- 1 ("Currently On")
      }
      frame "Set Measurement Conditions" {
        n207 = local read "Currently On"() -> (w540:i32)
        n208 = Decrement(x=w540) -> (x-1=w551:i32)
        n209 = Index Array(array=w552, index (row)=w551) -> (element=w550:dbl[])  [unwired: 1 in]
        n210 = case shown="\"Concentration\"" w539 {
          tunnel: w550 -> [w568 w585 w602]
          tunnel: w548 -> [_ _ w600]
          tunnel: w553 -> [w566 w581 w591]
          tunnel: [w567 w580 w589] -> w534
          tunnel: w540 -> [w562 _ w592]
          tunnel: [w565 w579 w596] -> w532
          frame "Tunnel Speed" {
            n211 = Index Array(array=w568, index=0 ("Index")) -> (element=w555:dbl)
            n212 = while {
              shift-right: [w576] -> w557
              shift-left: _ -> [w575]
              tunnel: w555 -> [w578]
              tunnel: [w576] -> w564
              tunnel: [w575] -> w563
              stop <- FALSE continue-if-true
              n213 = Greater Than 0?(x=w578) -> (x > 0?=w576:bool)
            }
            n214 = Exclusive Or(1:w563, 2:w564) -> (0:w560:bool)
            n215 = Greater?(x=w562, y=1) -> (0:w559:bool)
            n216 = And(x=w560, y=w559) -> (x .and. y?=w558:bool)
            n217 = case shown="False" w557 {
              tunnel: [w570 w572] -> w556
              tunnel: w555 -> [w571 w572]
              frame False {
                n218 = Negate(x=w571) -> (-x=w570:dbl)
              }
              frame True {
              }
            }
            n219 = case shown="True" w558 {
              frame False {
              }
              frame True {
                n220 = call "Wait_Seconds_with_display.vi"("Message"="Please rotate the probe you are calibrating", "Seconds to wait"=10000.0) -> ()  [unwired: 2 out]
              }
            }
            n221 = local read "Establishment time"() -> (w565:string)
            n222 = Bundle By Name(cluster=w566, "Tunnel Speed"=w556) -> (w567:T5)
          }
          frame "Traverse Position" {
            n223 = Index Array(array=w585, index=0 ("Index")) -> (element=w584:dbl)
            n224 = Index Array(array=w585, index=1 ("Index")) -> (element=w583:dbl)
            n225 = Index Array(array=w585, index=2 ("Index")) -> (element=w582:dbl)
            n226 = local read "Establishment time"() -> (w579:string)
            n227 = Bundle By Name(cluster=w581, "Start X"=w584, "Start Y"=w583, "Start Z"=w582) -> (w580:T5)
          }
          frame "Concentration" {
            w590 = nan ("Start X")
            n228 = local read "Wait factor"() -> (w595:dbl)
            n229 = Index Array(array=w602, index=0 ("Index")) -> (element=w593:dbl)
            n230 = case shown="1, Default" w592 {
              tunnel: [w604 w612 100.0] -> w594
              tunnel: w595 -> [w610 w613 _]
              frame 1, Default {
                n231 = local read "Time FFID valve moved"() -> (w607:dbl)
                n232 = Get Date/Time In Seconds() -> (seconds since 1Jan1904=w609:timestamp)
                n233 = Multiply(x=w610, y=35.0) -> (x*y=w606:dbl)
                n234 = To Double Precision Float(number=w609) -> (double precision float=w608:dbl)
                n235 = Subtract(x=w608, y=w607) -> (x-y=w605:dbl)
                n236 = Subtract(x=w606, y=w605) -> (x-y=w604:dbl)
              }
              frame 2 {
                n237 = Multiply(x=w613, y=25.0) -> (x*y=w612:dbl)
              }
              frame 3 {
              }
            }
            n238 = case shown="\"Check VI only\"" w600 {
              tunnel: w593 -> [w617 w618]
              tunnel: [w616 w619] -> w601
              frame "Check VI only" {
                n239 = To Long Integer(number=w617) -> (32bit integer=w616:i32)
              }
              frame "Run VI" {
                n240 = call "Fast_FID_Valve_Control.vi"("Requested Position"=w618) -> ("Achieved Posn."=w619:T22)  [unwired: 6 out]
              }
            }
            n241 = Number To Decimal String(number=w594) -> (decimal integer string=w597:string)  [unwired: 1 out]
            n242 = Concatenate Strings("!Establish Exp Conditions (s) = " ("Message"), w597) -> (w596:string)
            n243 = To Double Precision Float(number=w601) -> (double precision float=→"Valve position":dbl)
            n244 = Bundle By Name(cluster=w591, "Start X"=w590, "Start Y"=w590, "Start Z"=w590) -> (w589:T5)
          }
        }
        n245 = call "Add_Extra_Command.vi"("Traverse line"=w534, "Extra Command"=w532) -> ("Traverse line Out"=w533:T5)
        n246 = call "Set_Measurement_Conditions.vi"("Simulate/Run"=w548, "Currently on Point"=1, "Traverse line"=w533) -> ("Status Cluster"=w538:T21)  [unwired: 2 out]
        n247 = Unbundle By Name(w538) -> ("Status"=w537:T2)
        "Status" <- w537
        n248 = Equal?(x=w537, y=Multi_Run_Status."Continue" ("Status")) -> (x = y?=w544:bool)
        n249 = Equal?(x=User_Specific_mode."Run VI" ("Mode"), y=w548) -> (x = y?=w545:bool)
        n250 = Increment(x=w535) -> (x+1=w542:T1)
        n251 = And(x=w544, y=w545) -> (x .and. y?=w543:bool)
        n252 = Select(t=w535, s=w543, f=w542) -> (s? t:f=w541:T1)
      }
      frame "Measure Calibration Point" {
        n253 = case shown="\"Concentration\"" w626 {
          tunnel: w625 -> [_ w635]
          tunnel: [w629 w634] -> w621
          tunnel: [w627 w633] -> w620
          frame "Tunnel Speed", Default {
            n254 = local read "New Calib Filenames"() -> (w630:path[])
            n255 = Index Array(array=w630, index=0 ("Index")) -> (element=w631:path)
            n256 = call "Calibration.vi"("Mode"=Calib_mode."Take a New Calibration Point", "Calib file"=w631) -> ("Coefficients"=w627:dbl[][], "Status Out"=w629:T2)  [unwired: 1 in, 15 out]
          }
          frame "Concentration" {
            # "St Dev"
            # "Mean"
            n257 = stacked-sequence {
              seq-local: [_ w639 _] -> [_ _ w684]
              seq-local: [_ w638 _] -> [_ _ w683]
              tunnel: w635 -> [_ w642 _]
              tunnel: [_ w640 _] -> w634
              tunnel: [_ _ w685] -> w633
              frame #0 {
                n258 = global write "Meas_global.vi" "Remote control"(TRUE ("Remote control")) -> ()
                n259 = global write "Meas_global.vi" "Raw data option"(enum16{"Save raw data", "Raw data not saved"}."Save raw data" ("Raw data option")) -> ()
              }
              frame #1 {
                n260 = local read "New Calib Filenames"() -> (w643:path[])
                n261 = Index Array(array=w643, index=0 ("Index")) -> (element=w641:path)
                n262 = while {
                  tunnel: [w651] -> w640
                  tunnel: w641 -> [w650]
                  tunnel: w642 -> [w648]
                  tunnel: [w647] -> w639
                  tunnel: [w646] -> w638
                  i -> [w645]
                  stop <- w649 continue-if-true
                  n263 = stacked-sequence {
                    seq-local: [_ w653 _ _] -> [_ _ _ w677]
                    seq-local: [_ _ w662 _] -> [_ _ _ w681]
                    tunnel: [_ w653 _ _] -> w651
                    tunnel: w650 -> [_ w658 _ _]
                    tunnel: [_ _ _ w672] -> w649
                    tunnel: w648 -> [_ w654 _ _]
                    tunnel: [_ _ w663 _] -> w647
                    tunnel: [_ _ w662 _] -> w646
                    tunnel: w645 -> [_ _ _ w679]
                    frame #0 {
                      n264 = global write "Meas_global.vi" "Remote control"(TRUE ("Remote control")) -> ()
                    }
                    frame #1 {
                      n265 = call "Get_Data_Base_file_code.vi"("Results Filename"=w658, "Data Type"="Raw_Calibrations") -> ("Raw Data File Name"=w655:path)  [unwired: 3 out]
                      n266 = call "Measurement.vi"("setup"=Setup."Run Program", "Post Process"=Post_Process."Take New Data", "File"=Save_Data."Save No Data", "Raw data file"=w655, "Setup filename"=w654) -> ("Status Out"=w653:T2)  [unwired: 2 in, 12 out]
                    }
                    frame #2 {
                      n267 = local read "FF Indexes"() -> (w664:i16[])
                      n268 = global read "Meas_global.vi" "Time Trace"() -> (w661:T23[])
                      n269 = for {
                        tunnel: w664 -> [w671] mode=indexing
                        tunnel: [w670] -> w663 mode=indexing
                        tunnel: [w669] -> w662 mode=indexing
                        tunnel: w661 -> [w667]
                        n270 = Index Array(array=w667, index=w671) -> (element=w666:T23)
                        n271 = Unbundle By Name(w666) -> ("Eng Values"=w665:dbl[])
                        n272 = call "De-spiked_Stats.vi"("Raw Signal"=w665, "No of st dev to chop at"=6.0) -> ("mean"=w670:dbl, "standard deviation"=w669:dbl)  [unwired: 1 out]
                      }
                    }
                    frame #3 {
                      n273 = Greater?(x=w681, y=0.15) -> (0:w680:bool[])
                      n274 = Or Array Elements(Boolean array=w680) -> (logical OR=w674:bool)
                      n275 = Less?(x=w679, y=2) -> (x < y?=w675:bool)
                      n276 = Equal?(x=w677, y=Multi_Run_Status."Continue" ("Status Out")) -> (x = y?=w673:bool)
                      n277 = Compound Arithmetic op=AND(w673, w674, w675) -> (w672:bool)
                    }
                  }
                }
              }
              frame #2 {
                n278 = local read "FFID St Dev"() -> (w688:dbl[][])
                n279 = local read "Valve position"() -> (w692:dbl)
                n280 = local read "Concentrations"() -> (w686:dbl[])
                n281 = global read "Meas_global.vi" "Temp"() -> (w693:dbl)
                n282 = Build Array (concatenate)(w684, w683) -> (w687:dbl[])
                n283 = Build Array (concatenate)(w688, w687) -> (→"FFID St Dev":dbl[][])
                n284 = Index Array(array=w686, index=w692) -> (element=w691:dbl)
                n285 = local read "New Calib Filenames"() -> (w690:path[])
                n286 = for {
                  tunnel: w684 -> [w699] mode=indexing
                  tunnel: w693 -> [w698]
                  tunnel: w691 -> [w697]
                  tunnel: [w696] -> w685 mode=indexing
                  tunnel: w690 -> [w695] mode=indexing
                  tunnel: w683 -> [w694] mode=indexing
                  n287 = stacked-sequence {
                    tunnel: w699 -> [w705 _]
                    tunnel: w698 -> [w702 _]
                    tunnel: w697 -> [w704 _]
                    tunnel: [_ w707] -> w696
                    tunnel: w695 -> [_ w706]
                    tunnel: w694 -> [w700 _]
                    frame #0 {
                      n288 = Build Array(w704, w705, w700, 0.0 ("element"), w702) -> (w703:dbl[])
                      n289 = global write "Calib_global.vi" "Calibration Points"(w703) -> ()
                    }
                    frame #1 {
                      n290 = call "Calibration.vi"("Mode"=Calib_mode."Refit Curve", "Calib file"=w706) -> ("Coefficients"=w708:dbl[][])  [unwired: 1 in, 16 out]
                      n291 = Index Array(array=w708, index (row)=0 ("Index")) -> (element=w707:dbl[])  [unwired: 1 in]
                    }
                  }
                }
              }
            }
          }
        }
        "Coefficients" <- w620
        n292 = local write "Status"(w621) -> ()
      }
      frame "Do Another Calibration Point?" {
        n293 = local read "Status"() -> (w720:T2)
        n294 = local read "No of Calib Points"() -> (w724:i32)
        n295 = local read "Currently On"() -> (w716:i32)
        n296 = case shown="\"Terminate Run\"" w720 {
          tunnel: [w734 w735 TRUE w738] -> w722
          tunnel: [w734 w735 FALSE w738] -> w723
          frame "Continue", Default {
            w734 = TRUE
          }
          frame "Jump to Next Point" {
            w735 = TRUE
          }
          frame "Jump to Next Row" {
          }
          frame "Terminate Run" {
            w738 = FALSE
          }
        }
        n297 = Greater?(x=w724, y=w716) -> (0:w721:bool)
        n298 = Compound Arithmetic op=AND(invert "stop", w722) -> (w719:bool)
        n299 = Compound Arithmetic op=AND(w719, w723, w721) -> (w717:bool)
        n300 = case shown="False" w717 {
          tunnel: w716 -> [_ w733]
          tunnel: [w727 Auto_Calib_Case."Set Measurement Conditions" ("Currently in Case")] -> w715
          tunnel: w714 -> [w728 _]
          tunnel: w713 -> [w726 _]
          frame False {
            n301 = case shown="\"Check VI only\"" w728 {
              tunnel: [Auto_Calib_Case."End" ("Currently in Case") Auto_Calib_Case."Skip Next Frame?" ("Currently in Case")] -> w727
              tunnel: w726 -> [_ _]
              frame "Check VI only" {
              }
              frame "Run VI" {
              }
            }
          }
          frame True {
            n302 = Increment(x=w733) -> (x+1=w732:i32)
            n303 = local write "Currently On"(w732) -> ()
          }
        }
        n304 = case shown="True" "stop" {
          frame False {
          }
          frame True {
            n305 = local write "Status"(Multi_Run_Status."Terminate Run" ("Status")) -> ()
          }
        }
      }
      frame "Skip Next Frame?" {
        n306 = local read "Status"() -> (w742:T2)
        n307 = case shown="\"Tunnel Speed\", Default" w739 {
          frame "Tunnel Speed", Default {
          }
          frame "Concentration" {
            n308 = call "Fast_FID_Valve_Control.vi"("Requested Position"=4 ("Requested Posn.")) -> ()  [unwired: 7 out]
          }
        }
        n309 = case shown="\"Continue\"" w742 {
          tunnel: [w746 Auto_Calib_Case."End" ("Currently in Case")] -> w741
          tunnel: w740 -> [w746 _]
          frame "Continue" {
          }
          frame "Terminate Run", Default {
          }
        }
      }
      frame "Insert New calibration Filenames into Measurement Setup file" {
        n310 = local read "New Calib Filenames"() -> (w748:path[])
        n311 = global read "Meas_global.vi" "Raw data file"() -> (w758:path)
        n312 = local read "Ch No's"() -> (w749:i16[])
        n313 = Strip Path(path=w758) -> (stripped path=w757:path)  [unwired: 1 out]
        n314 = Equal?(x=Auto_Calib_Type."Concentration" ("Calibration varying"), y=w755) -> (x = y?=w754:bool)
        n315 = call "Current_Calib_Filenames.vi"("Calib Filename"=w748, "Channel Numbers"=w749, "Mode"=App_Global."Write to Global") -> ()  [unwired: 3 out]
        n316 = case shown="False" w754 {
          tunnel: [Auto_Calib_Case."Warn if Current Calibration fit is poor" ("Currently in Case") w765] -> w753
          tunnel: w752 -> [_ w765]
          tunnel: w748 -> [_ w764]
          tunnel: [1 w763] -> w751
          frame False {
          }
          frame True {
            n317 = Array Size(array=w764) -> (size(s)=w763:i32)
          }
        }
        n318 = for {
          N: w751 -> [_]
          tunnel: w748 -> [w767] mode=indexing
          tunnel: w757 -> [w771]
          w769 = FALSE  # Variable Target?
          n319 = Strip Path(path=w767) -> (name=w770:string)  [unwired: 1 out]
          n320 = Build Path(base path=w771, name or relative path=w770) -> (appended path=w766:path)
          n321 = call "Remember_Calib_Filenames.vi"("Filename to Remember"=w766) -> ()  [unwired: 1 out]
          n322 = call "Copy_with_Check.vi"("Mode"=enum16{"Move", "Copy"}."Copy", "Target Path"=w766, "Variable Target?"=w769, "Source Path"=w767) -> ()  [unwired: 1 out]
        }
      }
      frame "Warn if FFID calibration is very non linear" {
        w788 = FALSE  # Dialog Box (T)
        n323 = local read "Root Name"() -> (w787:string[])
        n324 = local read "Coefficients"() -> (w790:dbl[][])
        n325 = for {
          tunnel: w790 -> [w797] mode=indexing
          shift-right: [w799] -> w785
          shift-left: "" -> [w800]
          tunnel: w787 -> [w801] mode=indexing
          tunnel: [w794] -> w780 mode=indexing
          tunnel: "If the calibration fit for %s had been linear instead of a second order polynomial, it would have yielded an average fit error of %.1f%%.\\n" ("Format String") -> [w792]
          n326 = Index Array(array=w797, index=0 ("Index")) -> (element=w795:dbl)
          n327 = Absolute Value(x=w795) -> (abs(x)=w794:dbl)
          n328 = Less?(x=w794, y=2.2) -> (x < y?=w798:bool)
          n329 = case shown="False" w798 {
            tunnel: w801 -> [w803 _]
            tunnel: w794 -> [w804 _]
            tunnel: w800 -> [w807 w808]
            tunnel: [w805 w808] -> w799
            tunnel: w792 -> [w802 _]
            frame False {
              n330 = Format Into String(format string=w802, w803, w804) -> (resulting string=w806:string)  [unwired: 2 in, 1 out]
              n331 = Concatenate Strings(w807, w806) -> (w805:string)
            }
            frame True {
            }
          }
        }
        n332 = Array Max & Min(array=w780) -> (max value=w779:dbl)  [unwired: 3 out]
        n333 = Greater?(x=w779, y=7.0) -> (0:w777:bool)
        n334 = Select(t="Very Poor FFID Linearity", s=w777, f="Poor FFID Linearity") -> (s? t:f=w774:string)
        n335 = Empty String/Path?(string/path=w785) -> (empty?=w784:bool)
        n336 = Not(x=w784) -> (.not. x?=w783:bool)
        n337 = Bundle By Name(cluster=errorcluster {"status"=FALSE, "code"=0, "source"=""} ("error in (no error)"), "source"=w785, "status"=w783) -> (w782:errorcluster)
        n338 = call "EnFlo_Error_Handler.vi"("error in (no error)"=w782, "Error Type"=w774, "Dialog Box (T)"=w788) -> ()  [unwired: 3 out]
      }
      frame "Warn if FFID variance is high" {
        w830 = FALSE  # Dialog Box (T)
        n339 = local read "New Calib Filenames"() -> (w812:path[])
        n340 = local read "FFID St Dev"() -> (w832:dbl[][])
        n341 = Index Array(array=w817, index (col)=0 ("disabled index (col)")) -> (element=w815:dbl[])  [unwired: 1 in]
        n342 = Array Size(array=w812) -> (size(s)=w811:i32)
        n343 = for {
          tunnel: w832 -> [w849]
          shift-right: [w851] -> w828
          shift-left: "" -> [w852]
          tunnel: w812 -> [w840] mode=indexing
          tunnel: "For %s the measurement at %dppm had a standard deviation of %.2f volts for an average value of  %.1f volts.\\n" ("Format String") -> [w850]
          tunnel: w815 -> [w843]
          tunnel: [w842] -> w813 mode=indexing
          tunnel: w811 -> [w838]
          tunnel: [w834] -> w809 mode=indexing
          i -> [w837]
          n344 = Add(x=w838, y=w837) -> (x+y=w836:i32)
          n345 = Strip Path(path=w840) -> (name=w839:string)  [unwired: 1 out]
          n346 = Index Array(array=w849, index (col)=w837) -> (element=w841:dbl[])  [unwired: 1 in]
          n347 = Index Array(array=w849, index (col)=w836) -> (element=w835:dbl[])  [unwired: 1 in]
          n348 = Array Max & Min(array=w835) -> (min value=w834:dbl)  [unwired: 3 out]
          n349 = call-poly <vilib>:"Mean.vi"("X"=w841) -> ("mean"=w848:dbl)  [unwired: 1 out]
          n350 = Divide(x=w835, y=w848) -> (x/y=w847:dbl[])
          n351 = Array Max & Min(array=w847) -> (max value=w842:dbl, max index (indices)=w844:i32)  [unwired: 2 out]
          n352 = Greater?(x=w842, y=0.06) -> (0:w845:bool)
          n353 = case shown="True" w845 {
            tunnel: w839 -> [_ w863]
            tunnel: w852 -> [w853 w869]
            tunnel: [w853 w867] -> w851
            tunnel: w850 -> [_ w866]
            tunnel: w844 -> [_ w864]
            tunnel: w843 -> [_ w865]
            tunnel: w842 -> [_ _]
            tunnel: w835 -> [_ w862]
            tunnel: w841 -> [_ w860]
            frame False {
            }
            frame True {
              n354 = local read "Concentrations"() -> (w858:dbl[])
              n355 = Index Array(array=w865, index=w864) -> (element=w859:dbl)
              n356 = Index Array(array=w862, index=w864) -> (element=w856:dbl)
              n357 = Index Array(array=w860, index=w864) -> (element=w861:dbl)
              n358 = Index Array(array=w858, index=w859) -> (element=w857:dbl)
              n359 = Multiply(x=w856, y=2.5) -> (x*y=w855:dbl)
              n360 = Format Into String(format string=w866, w863, w857, w855, w861) -> (resulting string=w868:string)  [unwired: 2 in, 1 out]
              n361 = Concatenate Strings(w869, w868) -> (w867:string)
            }
          }
        }
        "Minimum St Dev" <- w809
        n362 = Array Max & Min(array=w813) -> (max value=w823:dbl)  [unwired: 3 out]
        n363 = Greater?(x=w823, y=0.09) -> (0:w821:bool)
        n364 = Select(t="Very unstable FFID calibration point", s=w821, f="Unstable FFID calibration point") -> (s? t:f=w818:string)
        n365 = Empty String/Path?(string/path=w828) -> (empty?=w827:bool)
        n366 = Not(x=w827) -> (.not. x?=w826:bool)
        n367 = Bundle By Name(cluster=errorcluster {"status"=FALSE, "code"=0, "source"=""} ("error in (no error)"), "source"=w828, "status"=w826) -> (w825:errorcluster)
        n368 = call "EnFlo_Error_Handler.vi"("error in (no error)"=w825, "Error Type"=w818, "Dialog Box (T)"=w830) -> ()  [unwired: 3 out]
      }
      frame "Insert Bkgnd Variance into calib file" {
        n369 = local read "New Calib Filenames"() -> (w872:path[])
        n370 = local read "Minimum St Dev"() -> (w873:dbl[])
        n371 = local read "Coefficients"() -> (w870:dbl[][])
        n372 = for {
          tunnel: w873 -> [w878] mode=indexing
          tunnel: w872 -> [w884] mode=indexing
          tunnel: w870 -> [w881] mode=indexing
          n373 = call "Read_File_Simple.vi"("Filename"=w884) -> ("string"=w888:string)  [unwired: 2 in, 7 out]
          n374 = Index Array(array=w881, index=2) -> (element=w879:dbl)
          n375 = Multiply(x=w878, y=w879) -> (x*y=w877:dbl)
          n376 = Square(x=w877) -> (x^2=w876:dbl)
          n377 = Number To Fractional String(number=w876, precision (6)=i16 8) -> (F-format string=w886:string)  [unwired: 2 out]
          n378 = call "Replace_data_in_setup_string.vi"("New data string"=w886, "Input string"=w888, "Variable name"="Fast FID Bkgnd Variance") -> ("Appended string"=w883:string)
          n379 = call "Write_File_Simple.vi"("append to file? (new file:F)"=FALSE, "character string"=w883, "file path"=w884) -> ()  [unwired: 2 out]
        }
      }
      frame "Warn if FFID voltages are too low" {
        w906 = FALSE  # Dialog Box (T)
        n380 = local read "Coefficients"() -> (w896:dbl[][])
        n381 = local read "Concentrations"() -> (w892:dbl[])
        n382 = Index Array(array=w899, index (col)=0 ("disabled index (col)")) -> (element=w891:dbl[])  [unwired: 1 in]
        n383 = local read "New Calib Filenames"() -> (w895:path[])
        n384 = for {
          tunnel: w892 -> [w911]
          tunnel: w891 -> [w910] mode=indexing
          tunnel: [w909] -> w890 mode=indexing
          n385 = Index Array(array=w911, index=w910) -> (element=w909:dbl)
        }
        n386 = Array Max & Min(array=w890) -> (max value=w889:dbl)  [unwired: 3 out]
        n387 = for {
          shift-right: [w921] -> w904
          shift-left: "" -> [w922]
          tunnel: "For %s the maximum measured calibration voltage was %.1f volts.\nCheck that the FID is running and correctly connected to the acquisition system." ("Format String") -> [w920]
          tunnel: w896 -> [w918] mode=indexing
          tunnel: w895 -> [w914] mode=indexing
          tunnel: w889 -> [w913]
          n388 = Split 1D Array(array=w918, index=1) -> (second subarray=w917:dbl[])  [unwired: 1 out]
          n389 = call "Polybackwards.vi"("Coefficients"=w917, "Y input"=w913) -> ("X output"=w912:dbl)  [unwired: 1 out]
          n390 = Less?(x=w912, y=0.2) -> (x < y?=w915:bool)
          n391 = case shown="True" w915 {
            tunnel: w922 -> [w923 w930]
            tunnel: [w923 w928] -> w921
            tunnel: w920 -> [_ w927]
            tunnel: w914 -> [_ w926]
            tunnel: w912 -> [_ w924]
            frame False {
            }
            frame True {
              n392 = Strip Path(path=w926) -> (name=w925:string)  [unwired: 1 out]
              n393 = Format Into String(format string=w927, w925, w924) -> (resulting string=w929:string)  [unwired: 2 in, 1 out]
              n394 = Concatenate Strings(w930, w929) -> (w928:string)
            }
          }
        }
        n395 = Empty String/Path?(string/path=w904) -> (empty?=w903:bool)
        n396 = Not(x=w903) -> (.not. x?=w902:bool)
        n397 = Bundle By Name(cluster=errorcluster {"status"=FALSE, "code"=0, "source"=""} ("error in (no error)"), "source"=w904, "status"=w902) -> (w901:errorcluster)
        n398 = call "EnFlo_Error_Handler.vi"("error in (no error)"=w901, "Error Type"="Low FFID calibration voltages", "Dialog Box (T)"=w906) -> ()  [unwired: 3 out]
      }
      frame "Warn if Current Calibration fit is poor" {
        w945 = FALSE  # Dialog Box (T)
        n399 = local read "Root Name"() -> (w944:string[])
        n400 = local read "Coefficients"() -> (w947:dbl[][])
        n401 = for {
          tunnel: w947 -> [w954] mode=indexing
          shift-right: [w956] -> w942
          shift-left: "" -> [w957]
          tunnel: w944 -> [w958] mode=indexing
          tunnel: [w951] -> w937 mode=indexing
          n402 = Index Array(array=w954, index=0 ("Index")) -> (element=w952:dbl)
          n403 = Absolute Value(x=w952) -> (abs(x)=w951:dbl)
          n404 = Less?(x=w951, y=1.0) -> (x < y?=w955:bool)
          n405 = case shown="True" w955 {
            tunnel: w958 -> [w960 _]
            tunnel: w951 -> [w961 _]
            tunnel: w957 -> [w964 w965]
            tunnel: [w962 w965] -> w956
            frame False {
              n406 = Format Into String(format string="The calibration for %s has an average fit error of %.1f%%\\n" ("Format String"), w960, w961) -> (resulting string=w963:string)  [unwired: 2 in, 1 out]
              n407 = Concatenate Strings(w964, w963) -> (w962:string)
            }
            frame True {
            }
          }
        }
        n408 = Array Max & Min(array=w937) -> (max value=w936:dbl)  [unwired: 3 out]
        n409 = Greater?(x=w936, y=7.0) -> (0:w934:bool)
        n410 = Select(t="Very Poor Calibration", s=w934, f="Poor Calibration") -> (s? t:f=w931:string)
        n411 = Empty String/Path?(string/path=w942) -> (empty?=w941:bool)
        n412 = Not(x=w941) -> (.not. x?=w940:bool)
        n413 = Bundle By Name(cluster=errorcluster {"status"=FALSE, "code"=0, "source"=""} ("error in (no error)"), "source"=w942, "status"=w940) -> (w939:errorcluster)
        n414 = call "EnFlo_Error_Handler.vi"("error in (no error)"=w939, "Error Type"=w931, "Dialog Box (T)"=w945) -> ()  [unwired: 3 out]
      }
      frame "Warn if Calibration Coefficients have significantly altered" {
        w991 = FALSE  # Dialog Box (T)
        w978 = 8.0 ("y")
        n415 = local read "New Calib Filenames"() -> (w983:path[])
        n416 = local read "Root Name"() -> (w982:string[])
        n417 = global read "Calib_global.vi" "Instrument type"() -> (w981:T14)
        n418 = Unbundle By Name(w970) -> ("Extra Commands"=w969:string)
        n419 = global read "Extra_Commands_Global.vi" "If Command"() -> (w971:string)
        n420 = call "Extra_Commands.vi"("String to Search"=w969, "Command"=w971) -> ("String Value"=w968:string)  [unwired: 1 in, 4 out]
        n421 = call "Calibration_Analysis.vi"("Root Name"=w982, "New Calib Filenames"=w983, "Instrument type"=w981, "Clear Calib History"="Clear Calib History") -> ("Error String"=w980:string, "Max % Error"=w966:dbl)
        n422 = call "Get_array_values_fr_String.vi"("String Value"=w968) -> ("Numeric Array"=w967:dbl[], "String array"=w973:string[])
        n423 = Greater?(x=w966, y=w978) -> (0:w979:bool)
        n424 = Index Array(array=w973, index=0 ("Index")) -> (element=w974:string)
        n425 = case shown="\"Drift Greater Than\"" w974 {
          tunnel: w967 -> [w997 _]
          tunnel: w966 -> [w996 _]
          frame "Drift Greater Than" {
            n426 = Index Array(array=w997, index=1 ("Index")) -> (element=w995:dbl)
            n427 = Greater?(x=w996, y=w995) -> (0:w994:bool)
            n428 = case shown="True" w994 {
              frame False {
              }
              frame True {
                n429 = local write "Status"(Multi_Run_Status."Jump To Fall Back" ("Status")) -> ()
              }
            }
          }
          frame "No Match", Default {
          }
        }
        n430 = Format Into String(format string="Calibration Drift Greater than %d%%", w978) -> (resulting string=w976:string)  [unwired: 2 in, 1 out]
        n431 = Select(t=w976, s=w979, f="Calibration Drift") -> (s? t:f=w984:string)
        n432 = Empty String/Path?(string/path=w980) -> (empty?=w989:bool)
        n433 = Not(x=w989) -> (.not. x?=w988:bool)
        n434 = Bundle By Name(cluster=errorcluster {"status"=FALSE, "code"=0, "source"=""} ("error in (no error)"), "source"=w980, "status"=w988) -> (w987:errorcluster)
        n435 = call "EnFlo_Error_Handler.vi"("error in (no error)"=w987, "Error Type"=w984, "Dialog Box (T)"=w991) -> ()  [unwired: 3 out]
      }
      frame "End" {
        n436 = local read "Original Calib File"() -> (w1004:path)
        n437 = Bundle By Name(cluster=w1001, "Filename"=w1004) -> ()  [unwired: 1 out]
        n438 = case shown="\"Concentration\"" w1003 {
          tunnel: w1001 -> [_ w1021]
          tunnel: w1002 -> [_ w1009]
          tunnel: w1000 -> [_ w1020]
          frame "Tunnel Speed", Default {
          }
          frame "Concentration" {
            n439 = Unbundle By Name(w1021) -> ("Averaging time (min)"=w1023:dbl)
            n440 = global read "Trav_pos_global.vi" "Simulation Time"() -> (w1012:timestamp)
            n441 = Unbundle By Name(w1021) -> ("Start Z"=w1008:dbl)
            n442 = Select(t=3 ("No. of pts."), s=w1020, f=2 ("No. of pts.")) -> (s? t:f=w1014:i32)
            n443 = Multiply(x=60.0, y=w1023) -> (x*y=w1017:dbl)
            n444 = Add(x=w1008, y=50.0) -> (x+y=w1024:dbl)
            n445 = Add(x=w1017, y=60.0) -> (x+y=w1015:dbl)
            n446 = Bundle By Name(cluster=w1021, "Start Z"=w1024) -> (w1025:T5)
            n447 = Multiply(x=w1015, y=w1014) -> (x*y=w1013:dbl)
            n448 = Add(x=w1012, y=w1013) -> (x+y=w1010:timestamp)
            n449 = call "Set_Traverse_Position.vi"("Simulate/Run"=w1009, "Currently on Point"=1, "Traverse line"=w1025) -> ()  [unwired: 3 out]
            n450 = call "Run_FFID_Bkgnd.vi"("Simulated Time"=w1010, "Run Now?"=TRUE, "Simulate/Run"=w1009) -> ()  [unwired: 3 out]
          }
        }
        "Traverse Out" <- w1001
      }
    }
    "Currently in Case" <- w10
  }
  "Error Messages" <- w5
